vi "Generate_3D_Mesh.vi"(8 "XYZ Input":cluster{"X":sgl, "Y":sgl, "Z":sgl}[](array[cluster]), 10 "Normal Binding Mode":T1(ring), 11 "Primitive Mode":T3(ring)) -> (1 "Normal Array":cluster{"X":sgl, "Y":sgl, "Z":sgl}[](array[cluster]), 2 "Indices":u32[](array[numeric]), 3 "Vertex Array":cluster{"X":sgl, "Y":sgl, "Z":sgl}[](array[cluster]), 4 "Texture Array":cluster{"X":sgl, "Y":sgl}[](array[cluster]), 5 "Color Array":T2(array[cluster]))   [LabVIEW 2016]
doc: "Create meshes of points for the Using Meshes.vi example. Define some known parameters so the mesh can be processed."
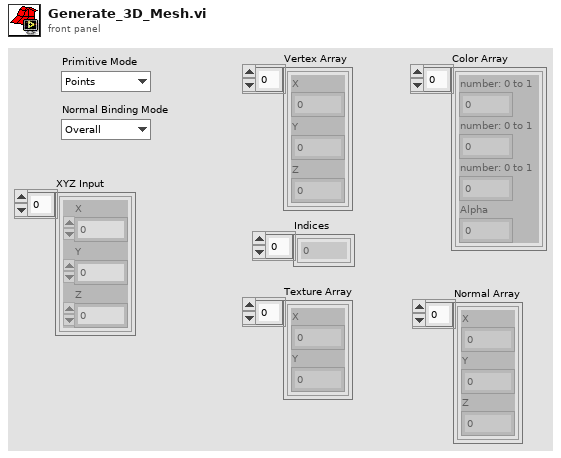
[diagram p1: front panel]
types:
  T1 = enum16{"Overall", "Per Primitive", "Per Vertex", "Binding Off"}
  T2 = cluster{"number: 0 to 1":dbl, "number: 0 to 1":dbl, "number: 0 to 1":dbl, "Alpha":dbl}[]
  T3 = enum16{"Points", "Lines", "Line Strip", "Line Loop", "Triangles", "Triangle Strip", "Triangle Fan", "Quads", "Quad Strip", "Polygon"}
  T4 = cluster{"number: 0 to 1":dbl, "number: 0 to 1":dbl, "number: 0 to 1":dbl}[]
  T5 = cluster{"number: 0 to 1":dbl, "number: 0 to 1":dbl, "number: 0 to 1":dbl, dbl}
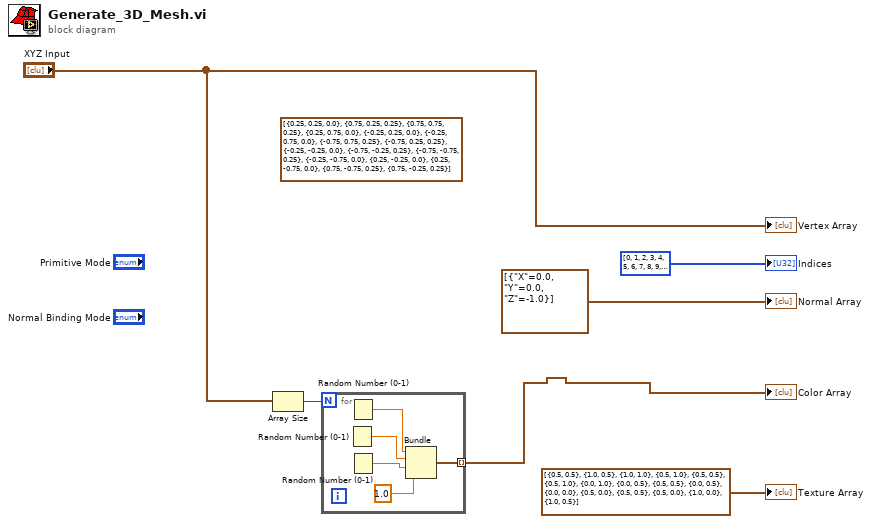
[diagram p0: block diagram]
diagram:
  (unwired) T4 [{"number: 0 to 1"=0.25, "number: 0 to 1"=0.25, "number: 0 to 1"=0.0}, {"number: 0 to 1"=0.75, "number: 0 to 1"=0.25, "number: 0 to 1"=0.25}, {"number: 0 to 1"=0.75, "number: 0 to 1"=0.75, "number: 0 to 1"=0.25}, {"number: 0 to 1"=0.25, "number: 0 to 1"=0.75, "number: 0 to 1"=0.0}, {"number: 0 to 1"=-0.25, "number: 0 to 1"=0.25, "number: 0 to 1"=0.0}, {"number: 0 to 1"=-0.25, "number: 0 to 1"=0.75, "number: 0 to 1"=0.0}, {"number: 0 to 1"=-0.75, "number: 0 to 1"=0.75, "number: 0 to 1"=0.25}, {"number: 0 to 1"=-0.75, "number: 0 to 1"=0.25, "number: 0 to 1"=0.25}, {"number: 0 to 1"=-0.25, "number: 0 to 1"=-0.25, "number: 0 to 1"=0.0}, {"number: 0 to 1"=-0.75, "number: 0 to 1"=-0.25, "number: 0 to 1"=0.25}, {"number: 0 to 1"=-0.75, "number: 0 to 1"=-0.75, "number: 0 to 1"=0.25}, {"number: 0 to 1"=-0.25, "number: 0 to 1"=-0.75, "number: 0 to 1"=0.0}, {"number: 0 to 1"=0.25, "number: 0 to 1"=-0.25, "number: 0 to 1"=0.0}, {"number: 0 to 1"=0.25, "number: 0 to 1"=-0.75, "number: 0 to 1"=0.0}, {"number: 0 to 1"=0.75, "number: 0 to 1"=-0.75, "number: 0 to 1"=0.25}, {"number: 0 to 1"=0.75, "number: 0 to 1"=-0.25, "number: 0 to 1"=0.25}] ("Vertex Array")
  n1 = Array Size(array="XYZ Input") -> (size(s)=w3:i32)
  n2 = for {
    N: w3 -> [_]
    tunnel: [w11] -> w1 mode=indexing
    n3 = Random Number (0-1)() -> (number: 0 to 1=w8:dbl)
    n4 = Random Number (0-1)() -> (number: 0 to 1=w9:dbl)
    n5 = Random Number (0-1)() -> (number: 0 to 1=w7:dbl)
    n6 = Bundle("number: 0 to 1"=w9, "number: 0 to 1"=w8, "number: 0 to 1"=w7, 1.0) -> (w11:T5)  [unwired: 1 in]
  }
  "Color Array" <- w1
  "Vertex Array" <- "XYZ Input"
  "Texture Array" <- cluster{"X":sgl, "Y":sgl}[] [{"X"=0.5, "Y"=0.5}, {"X"=1.0, "Y"=0.5}, {"X"=1.0, "Y"=1.0}, {"X"=0.5, "Y"=1.0}, {"X"=0.5, "Y"=0.5}, {"X"=0.5, "Y"=1.0}, {"X"=0.0, "Y"=1.0}, {"X"=0.0, "Y"=0.5}, {"X"=0.5, "Y"=0.5}, {"X"=0.0, "Y"=0.5}, {"X"=0.0, "Y"=0.0}, {"X"=0.5, "Y"=0.0}, {"X"=0.5, "Y"=0.5}, {"X"=0.5, "Y"=0.0}, {"X"=1.0, "Y"=0.0}, {"X"=1.0, "Y"=0.5}] ("Vertex Array")
  "Normal Array" <- cluster{"X":sgl, "Y":sgl, "Z":sgl}[] [{"X"=0.0, "Y"=0.0, "Z"=-1.0}]
  "Indices" <- u32[] [0, 1, 2, 3, 4, 5, 6, 7, 8, 9, 10, 11, 12, 13, 14, 15] ("Indices")
